vi "DLL 호출.vi"() -> ()   [LabVIEW 2014]
panel:
  out "array":dbl[](array[numeric])
  in  "경로":path
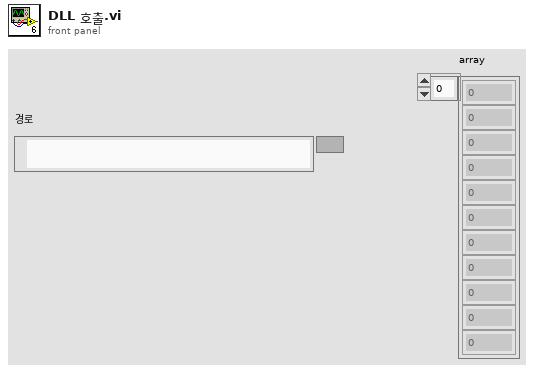
[diagram p1: front panel]
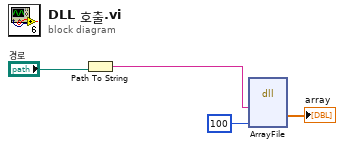
[diagram p0: block diagram]
diagram:
  n1 = Path To String(path="경로") -> (string=w3:string)
  n2 = dll-call lib="PTH2Jabs Cbuilds공유라이브러리만들기\n나의 DLL\nSharedLib.dll" fn="ArrayFile"("filePath"=w3, "len"=100) -> ("array"=→"array":dbl[])  [unwired: 7 in, 2 out]
